vi "Email Users.vi"() -> ()   [LabVIEW 2019]
uses:
  <vilib>/addons/database/Auxilliary.llb/DB Tools Cursor Type.ctl
  <vilib>/addons/database/Connection.llb/DB Tools Open Connec (String).vi
  <vilib>/addons/database/Connection.llb/Conn Execute.vi
  <vilib>/addons/database/Recordset.llb/Rec Fetch Recordset Data (R).vi
  <vilib>/addons/database/Recordset.llb/Rec Destroy - Connection.vi
  <vilib>/addons/database/_DB Variant To Data/Database Variant To Data.xnode
  <vilib>/addons/database/NI_Database_API.lvlib
panel:
  out "Messages Out":string[](array[string])
types:
  T1 = typedef "NI_Database_API.lvlib/DB Tools Cursor Type.ctl" = enum16{"forward-only", "keyset", "dynamic", "static"}
  T2 = typedef "NI_Database_API.lvlib/Conn ObjectReference.ctl" = refnum<k1>
  T3 = typedef "NI_Database_API.lvlib/Rec ObjectReference.ctl" = refnum<k1>
  T4 = typedef "Inventory Data Type.ctl" = cluster{"Identifier":string, "BYU ICN #":string, "Item Description":string, "Comments":string, "Checked Out Date":string, "Due Date":string, "Check Out Location":string, "Reminder Count":i32, "Most Recent Reminder Date":string, "BYU ID #":string, "Building/Room":string, "Location in Room":string, "Manual":string, "Manufacturer":string, "Model #":string, "Serial #":string, "Date Acquired":string, "Reminder Notes":string}
  T5 = cluster{"NOT DUE ITEMS":T4[], "DUE ITEMS":T4[], "REMINDER ITEMS":T4[], "EARLY REMINDER ITEMS":T4[]}
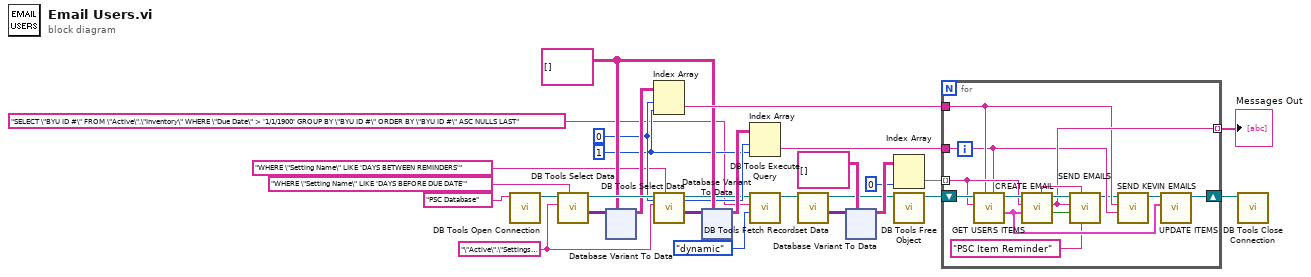
[diagram p0: block diagram]
diagram:
  w11 = 1 ("index (row)")
  w12 = 0 ("index (row)")
  w15 = string[][] []
  w17 = "\"Active\".\"Settings\"" ("table")
  n1 = call-poly <vilib>:"DB Tools Open Connection.vi"("connection information"="PSC Database") -> ("connection reference"=w21:T2)  [unwired: 7 in, 1 out]
  n2 = call <vilib>:"DB Tools Select Data.vi"("condition"="WHERE \"Setting Name\" LIKE 'DAYS BEFORE DUE DATE'", "table"=w17, "connection reference"=w21) -> ("data"=w19:variant[][], "connection reference out"=w18:T2)  [unwired: 3 in, 1 out]
  n3 = xnode "Database Variant To Data"("database variant"=w19, "type"=w15) -> ("data"=w14:string[][])  [unwired: 1 in, 1 out]
  n4 = Index Array(array=w14, index (row)=w12, index (col)=w11) -> (element=w27:string)
  n5 = call <vilib>:"DB Tools Select Data.vi"("condition"="WHERE \"Setting Name\" LIKE 'DAYS BETWEEN REMINDERS'", "table"=w17, "connection reference"=w18) -> ("data"=w16:variant[][], "connection reference out"=w10:T2)  [unwired: 3 in, 1 out]
  n6 = xnode "Database Variant To Data"("database variant"=w16, "type"=w15) -> ("data"=w13:string[][])  [unwired: 1 in, 1 out]
  n7 = Index Array(array=w13, index (row)=w12, index (col)=w11) -> (element=w26:string)
  n8 = call-poly <vilib>:"DB Tools Execute Query.vi"("cursor type"=DB_Tools_Cursor_Type."dynamic", "SQL query"="SELECT \"BYU ID #\" FROM \"Active\".\"Inventory\" WHERE \"Due Date\" > '1/1/1900' GROUP BY \"BYU ID #\" ORDER BY \"BYU ID #\" ASC NULLS LAST", "connection reference"=w10) -> ("recordset reference"=w22:T3)  [unwired: 5 in, 1 out]
  n9 = call-poly <vilib>:"DB Tools Fetch Recordset Data.vi"("recordset reference"=w22) -> ("recordset data"=w9:variant[][], "recordset reference out"=w2:T3)  [unwired: 4 in, 1 out]
  n10 = xnode "Database Variant To Data"("database variant"=w9, "type"=string[][] []) -> ("data"=w4:string[][])  [unwired: 1 in, 1 out]
  n11 = Index Array(array=w4, index (col)=0 ("disabled index (col)")) -> (element=w28:string[])  [unwired: 1 in]
  n12 = call-poly <vilib>:"DB Tools Free Object.vi"("recordset reference"=w2) -> ("connection reference"=w25:T2)  [unwired: 9 in, 1 out]
  n13 = for {
    tunnel: w28 -> [w40] mode=indexing
    shift-right: [w29] -> w24
    shift-left: w25 -> [w42]
    tunnel: w27 -> [w34]
    tunnel: w26 -> [w33]
    tunnel: [w35] -> w23 mode=indexing
    n14 = call "GET USERS ITEMS.vi"("DAYS BETWEEN REMINDERS"=w33, "DAYS BEFORE DUE DATE"=w34, "BYU ID # IN"=w40, "connection reference in"=w42) -> ("DATA OUT"=w36:T5, "connection reference out"=w41:T2)  [unwired: 6 in]
    n15 = call "CREATE EMAIL.vi"("DATA IN"=w36, "BYU ID # IN"=w40, "connection reference in"=w41) -> ("SEND EMAIL"=w38:bool, "MESSAGE OUT"=w35:string, "connection reference out"=w39:T2, "USER EMAIL OUT"=w37:string)  [unwired: 4 in, 1 out]
    n16 = call "SEND EMAILS.vi"("Subject"="PSC Item Reminder", "USER EMAIL IN"=w37, "SEND EMAIL"=w38, "MESSAGE IN"=w35, "connection reference in"=w39) -> ("connection reference out"=w31:T2)  [unwired: 6 in]
    n17 = call "SEND KEVIN EMAILS.vi"("DAYS BETWEEN REMINDERS"=w33, "DAYS BEFORE DUE DATE"=w34, "connection reference in"=w31) -> ("reference"=w30:T2)  [unwired: 8 in]
    n18 = call "UPDATE ITEMS.vi"("DATA IN"=w36, "connection reference in"=w30) -> ("connection reference out"=w29:T2)  [unwired: 9 in]
  }
  "Messages Out" <- w23
  n19 = call <vilib>:"DB Tools Close Connection.vi"("connection reference"=w24) -> ()  [unwired: 6 in, 1 out]
